vi "Create-Destroy.vi"(8 "Error In":errorcluster) -> (0 "Error Out":errorcluster)   [LabVIEW 2017, in "Tests.lvlib" / "KnownHosts.lvlib"]
uses:
  KnownHosts.lvlib
  src/LabSSH2/LabSSH2.lvlib
  src/LabSSH2/Public/Session/Session.lvclass
  <vilib>/addons/_JKI Toolkits/Caraya/classes/Test/Test.lvclass
  <vilib>/addons/_JKI Toolkits/Caraya/classes/Assert/Assert.lvclass
  src/LabSSH2/Public/KnownHosts/KnownHosts.lvclass
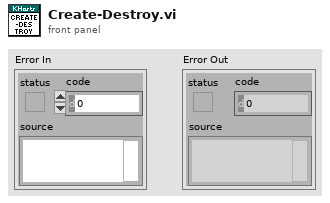
[diagram p1: front panel]
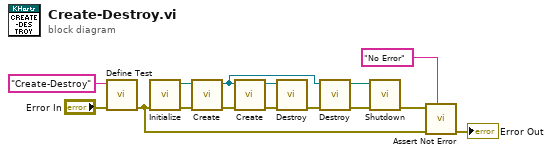
[diagram p0: block diagram]
diagram:
  n1 = call <vilib>:"Define Test.vi"("error in (no error)"="Error In", "Label (VI Title)"="Create-Destroy") -> ("error out"=w10:errorcluster)  [unwired: 9 in]
  n2 = call "Initialize.vi"("Error In"=w10) -> ("Error Out"=w14:errorcluster, "labssh2 Shared Library Out"=w6:path)  [unwired: 9 in]
  n3 = call "Create.vi"("Error In"=w14, "labssh2 Shared Library"=w6) -> ("Error Out"=w5:errorcluster, "Sesssion"=w1:refnum<class "Session.lvclass">)  [unwired: 8 in]
  n4 = call "Create.vi"("Error In"=w5, "Session"=w1) -> ("Error Out"=w3:errorcluster, "Known Hosts"=w4:refnum<class "KnownHosts.lvclass">)  [unwired: 8 in]
  n5 = call "Destroy.vi"("Error In"=w3, "KnownHosts"=w4) -> ("Error Out"=w2:errorcluster)  [unwired: 9 in]
  n6 = call "Destroy.vi"("Error In"=w2, "Session"=w1) -> ("Error Out"=w12:errorcluster, "labssh2 Shared Library"=w13:path)  [unwired: 8 in]
  n7 = call "Shutdown.vi"("Error In"=w12, "labssh2 Shared Library"=w13) -> ("Error Out"=w11:errorcluster)  [unwired: 9 in]
  n8 = call <vilib>:"Assert Not Error.vi"("Label"="No Error", "error in (no error)"=w10, "Not Error?"=w11) -> ("error out"=→"Error Out":errorcluster)  [unwired: 8 in]
